vi "Send UUT Detail Query.vi"(8 "error in":errorcluster, 11 "Launcher in":refnum<class "Launcher.lvclass">) -> (0 "error out":errorcluster, 2 "UUT Info":T1, 3 "Launcher out":refnum<class "Launcher.lvclass">)   [LabVIEW 2023, in "Launcher.lvlib" / "Launcher.lvclass"]
uses:
  Library/Launcher.lvclass
  Library/Launcher.lvclass/Launcher.ctl
  builds/Base Software/Base Software.lvlibp/Base Software Messages/Query UUT Details Msg/Query UUT Details Msg.lvclass
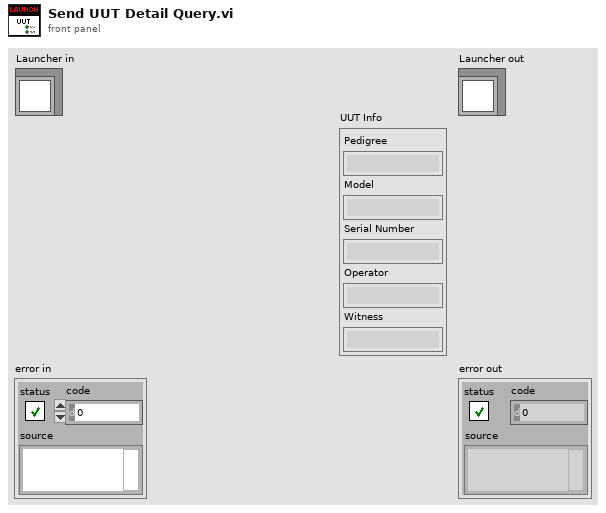
[diagram p1: front panel]
types:
  T1 = cluster{"Pedigree":string, "Model":string, "Serial Number":string, "Operator":string, "Witness":string}
  T2 = cluster{"[0]":string, "[1]":string, "[2]":string, "[3]":string, "[4]":string}
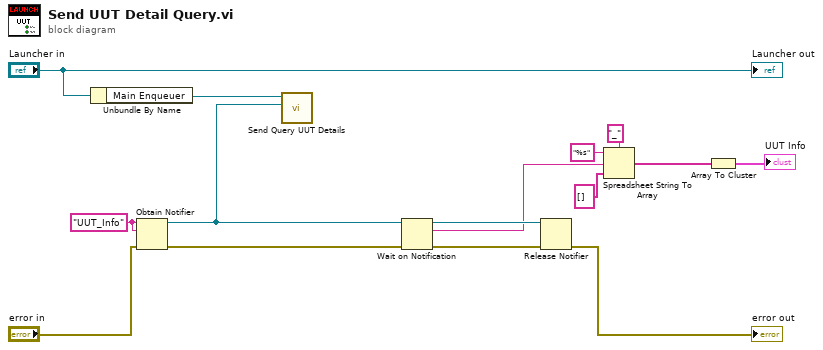
[diagram p0: block diagram]
diagram:
  w10 = "UUT_Info" ("name (unnamed)")
  n1 = Unbundle By Name("Launcher in") -> ("Main Enqueuer"=w2:refnum<class "Message Enqueuer.lvclass">)
  n2 = Obtain Notifier(name (unnamed)=w10, notification data type=w10, error in (no error)="error in") -> (notifier out=w1:refnum<notifier>, error out=w8:errorcluster)  [unwired: 1 in, 1 out]
  n3 = call "Send Query UUT Details.vi"("Name_Request"=w1, "Message Enqueuer"=w2) -> ()  [unwired: 8 in, 2 out]
  n4 = Wait on Notification(notifier=w1, error in (no error)=w8) -> (notifier out=w9:refnum<notifier>, notification=w4:string, error out=w7:errorcluster)  [unwired: 2 in, 1 out]
  n5 = Release Notifier(notifier=w9, error in (no error)=w7) -> (error out=→"error out":errorcluster)  [unwired: 1 in, 2 out]
  n6 = Spreadsheet String To Array(delimiter (Tab)="_", format string="%s", spreadsheet string=w4, array type (2D Dbl)=string[] []) -> (array=w11:string[])
  n7 = Array To Cluster(array=w11) -> (cluster=→"UUT Info":T2)
  "Launcher out" <- "Launcher in"
